vi "Get URI String.vi"(8 "error in (no error)":errorcluster, 11 "URI in":refnum<class "URI.lvclass">) -> (0 "error out":errorcluster, 2 "URI String":string, 3 "URI out":refnum<class "URI.lvclass">)   [LabVIEW 2020, in "IO.lvlib" / "URI.lvclass"]
uses:
  URI.lvclass
  URI.lvclass/URI.ctl
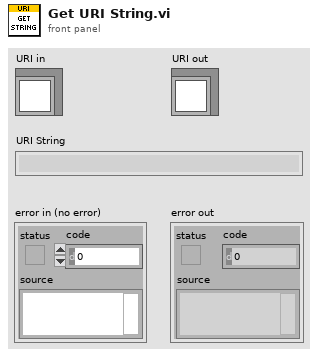
[diagram p1: front panel]
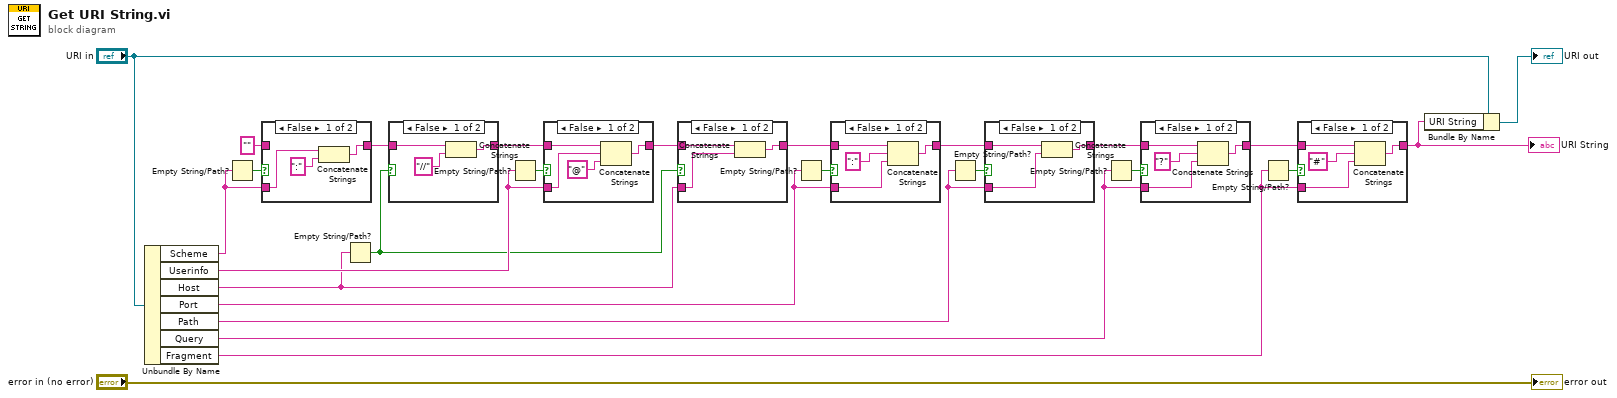
[diagram p0: block diagram]
diagram:
  n1 = Unbundle By Name("URI in") -> ("Scheme"=w24:string, "Userinfo"=w22:string, "Host"=w19:string, "Port"=w16:string, "Path"=w13:string, "Query"=w8:string, "Fragment"=w7:string)
  n2 = Empty String/Path?(string/path=w24) -> (empty?=w25:bool)
  n3 = case shown="False" w25 {
    tunnel: w24 -> [w29 _]
    tunnel: "" -> [_ w30]
    tunnel: [w27 w30] -> w2
    frame False {
      n4 = Concatenate Strings(w29, ":" ("string")) -> (w27:string)
    }
    frame True {
    }
  }
  n5 = Empty String/Path?(string/path=w19) -> (empty?=w1:bool)
  n6 = case shown="False" w1 {
    tunnel: w2 -> [w31 w34]
    tunnel: [w32 w34] -> w3
    frame False {
      n7 = Concatenate Strings(w31, "//" ("string")) -> (w32:string)
    }
    frame True {
    }
  }
  n8 = Empty String/Path?(string/path=w22) -> (empty?=w21:bool)
  n9 = case shown="False" w21 {
    tunnel: w22 -> [w38 _]
    tunnel: w3 -> [w35 w39]
    tunnel: [w36 w39] -> w20
    frame False {
      n10 = Concatenate Strings(w35, w38, "@" ("string")) -> (w36:string)
    }
    frame True {
    }
  }
  n11 = case shown="False" w1 {
    tunnel: w19 -> [w42 _]
    tunnel: w20 -> [w40 w43]
    tunnel: [w41 w43] -> w17
    frame False {
      n12 = Concatenate Strings(w40, w42) -> (w41:string)
    }
    frame True {
    }
  }
  n13 = Empty String/Path?(string/path=w16) -> (empty?=w18:bool)
  n14 = case shown="False" w18 {
    tunnel: w16 -> [w44 _]
    tunnel: w17 -> [w46 w48]
    tunnel: [w47 w48] -> w14
    frame False {
      n15 = Concatenate Strings(w46, ":" ("string"), w44) -> (w47:string)
    }
    frame True {
    }
  }
  n16 = Empty String/Path?(string/path=w13) -> (empty?=w15:bool)
  n17 = case shown="False" w15 {
    tunnel: w13 -> [w49 _]
    tunnel: w14 -> [w50 w52]
    tunnel: [w51 w52] -> w10
    frame False {
      n18 = Concatenate Strings(w50, w49) -> (w51:string)
    }
    frame True {
    }
  }
  n19 = Empty String/Path?(string/path=w8) -> (empty?=w11:bool)
  n20 = case shown="False" w11 {
    tunnel: w8 -> [w53 _]
    tunnel: w10 -> [w55 w57]
    tunnel: [w56 w57] -> w9
    frame False {
      n21 = Concatenate Strings(w55, "?" ("string"), w53) -> (w56:string)
    }
    frame True {
    }
  }
  n22 = Empty String/Path?(string/path=w7) -> (empty?=w12:bool)
  n23 = case shown="False" w12 {
    tunnel: w7 -> [w58 _]
    tunnel: w9 -> [w60 w62]
    tunnel: [w61 w62] -> w4
    frame False {
      n24 = Concatenate Strings(w60, "#" ("string"), w58) -> (w61:string)
    }
    frame True {
    }
  }
  "URI String" <- w4
  n25 = Bundle By Name(cluster="URI in", "URI String"=w4) -> (→"URI out":refnum<class "URI.lvclass">)
  "error out" <- "error in (no error)"
